vi "CAN Flatten.vi"(7 "payload in":u8[](array[numeric]), 8 "error in (no error)":errorcluster, 10 "Data in":u8[](array[numeric]) format="%.0x", 11 "CIFFifo in":refnum<class "CIFfifo.lvclass">) -> (0 "error out":errorcluster, 3 "CIFFifo out":refnum<class "CIFfifo.lvclass">, 5 "payload out":u8[](array[numeric]))   [LabVIEW 2021]
uses:
  CIFfifo.lvclass
  CIFfifo.lvclass/CIFfifo.ctl
  Accessors/Write Payload Length.vi
  Accessors/Read Header.vi
  <vilib>/CIF Foundation/CIF Utilities/DataTypes/Flatten U64.vi
  <vilib>/CIF Foundation/CIF Utilities/DataTypes/Flatten I64.vi
  ChannelCommon.lvlib
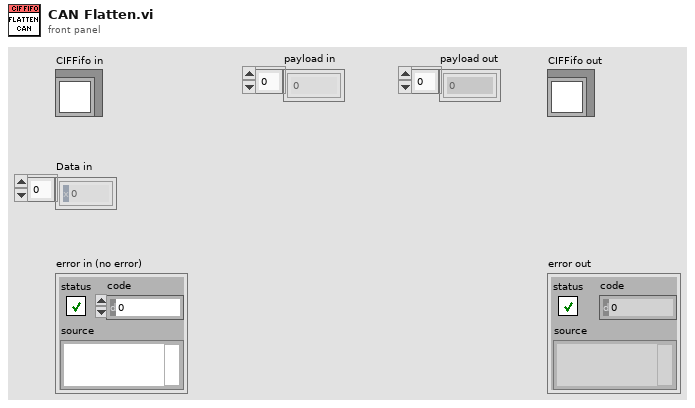
[diagram p1: front panel]
types:
  T1 = typedef "ChannelCommon.lvlib/FIFO Header.ctl" = cluster{"Length":u64, "T0":i64, "T_Out":i64, "T_Tx":i64, "Ctr":u64, "ClockID":u8}
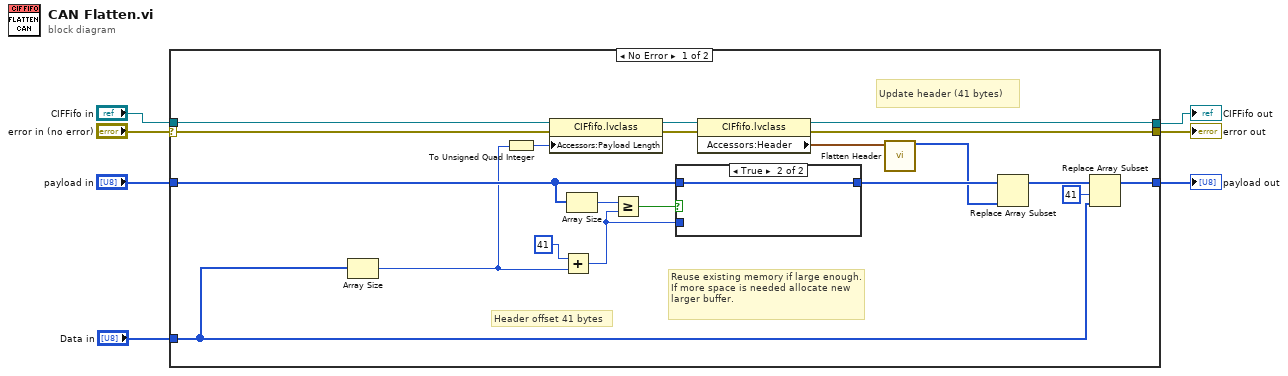
[diagram p0: block diagram]
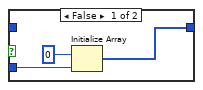
[diagram p2: hidden frame]
diagram:
  n1 = case shown="No Error" "error in (no error)" {
    selector: "error in (no error)" -> [w20 w34]
    tunnel: [w8 w34] -> w6
    tunnel: "CIFFifo in" -> [w27 w33]
    tunnel: [w17 w33] -> w2
    tunnel: [w9 w32] -> w4
    tunnel: "payload in" -> [w21 w32]
    tunnel: "Data in" -> [w11 _]
    frame No Error {
      # "Header offset 41 bytes"
      # "Update header (41 bytes)"
      # "Reuse existing memory if large enough.  If more space is needed allocate new larger buffer."
      n2 = Array Size(array=w11) -> (size(s)=w15:i32)
      n3 = To Unsigned Quad Integer(1:w15) -> (0:w25:u64)
      n4 = property class="CIFfifo.lvclass"(reference=w27, error in=w20, "Accessors:Payload Length"=w25) -> (reference out=w19:refnum<class "CIFfifo.lvclass">, error out=w18:errorcluster)
      n5 = Add(x=41 ("y"), y=w15) -> (x+y=w22:i32)
      n6 = Array Size(array=w21) -> (size(s)=w24:i32)
      n7 = Greater Or Equal?(x=w24, y=w22) -> (x >= y?=w23:bool)
      n8 = case shown="True" w23 {
        tunnel: w21 -> [_ w31]
        tunnel: [w28 w31] -> w14
        tunnel: w22 -> [w30 _]
        frame False {
          n9 = Initialize Array(u8 0, w30) -> (w28:u8[])
        }
        frame True {
        }
      }
      n10 = property class="CIFfifo.lvclass"(reference=w19, error in=w18) -> (reference out=w17:refnum<class "CIFfifo.lvclass">, error out=w8:errorcluster, "Accessors:Header"=w26:T1)
      n11 = call "Flatten Header.vi"("Header in"=w26) -> ("Flattened Data out"=w13:u8[])  [unwired: 10 in]
      n12 = Replace Array Subset(array=w14, new element=w13) -> (w12:u8[])  [unwired: 1 in]
      n13 = Replace Array Subset(array=w12, new element=w11, index=41) -> (w9:u8[])
    }
    frame Error {
    }
  }
  "error out" <- w6
  "CIFFifo out" <- w2
  "payload out" <- w4
